vi "evaluate_SP_thcd401_ch1.vi"(7 "PID Range":cluster{"output high":dbl, "output low":dbl}={"output high"=10.0, "output low"=-10.0} {"output low" format="%.2f"; "output high" format="%.2f"}, 8 "ref_sp_ch1":refnum<vi>, 10 "F_org":dbl, 11 "control":dbl) -> (0 "status":u32(colorbox), 3 "F_new":dbl)   [LabVIEW 2019]
panel:
  out "lolo":dbl
  out "hihi":dbl
  out "lo":dbl=22.0
  out "hi":dbl=38.0
  in  "range_error":dbl=0.95
  in  "range_warn":dbl=0.9
  # "L/m"
  # "L/m"
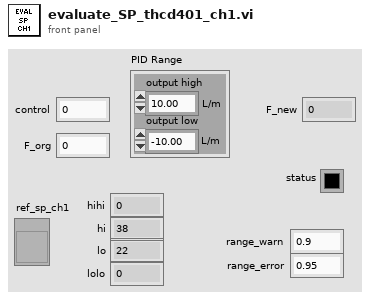
[diagram p1: front panel]
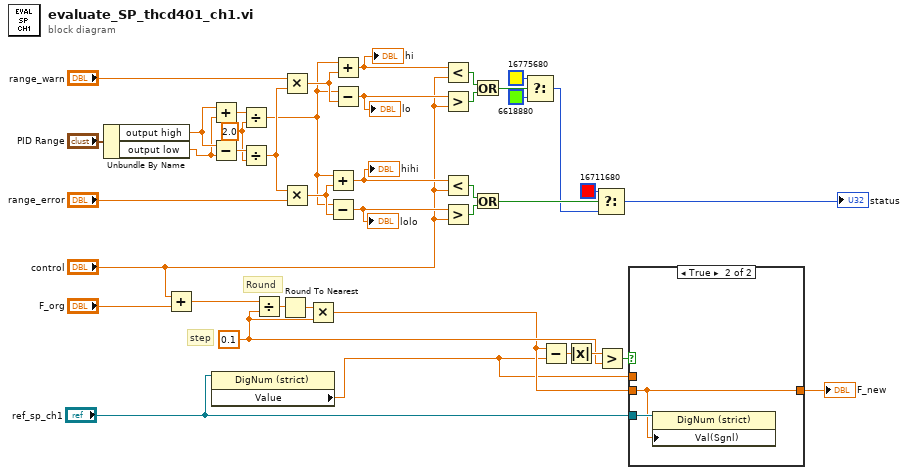
[diagram p0: block diagram]
diagram:
  w25 = 2.0 ("y")
  w34 = 0.1 ("y")
  # "Round"
  # "step"
  n1 = Unbundle By Name("PID Range") -> ("output high"=w20:dbl, "output low"=w19:dbl)
  n2 = Add(x="control", y="F_org") -> (x+y=w33:dbl)
  n3 = Add(x=w20, y=w19) -> (x+y=w27:dbl)
  n4 = Subtract(x=w20, y=w19) -> (x-y=w26:dbl)
  n5 = property class="DigNum (strict)"(reference="ref_sp_ch1") -> ("Value"=w3:dbl)  [unwired: 1 in, 2 out]
  n6 = Divide(x=w27, y=w25) -> (x/y=w10:dbl)
  n7 = Divide(x=w26, y=w25) -> (x/y=w11:dbl)
  n8 = Divide(x=w33, y=w34) -> (x/y=w36:dbl)
  n9 = Round To Nearest(number=w36) -> (nearest integer value=w35:dbl)
  n10 = Multiply(x="range_warn", y=w11) -> (x*y=w24:dbl)
  n11 = Multiply(x=w11, y="range_error") -> (x*y=w17:dbl)
  n12 = Multiply(x=w35, y=w34) -> (x*y=w9:dbl)
  n13 = Add(x=w10, y=w17) -> (x+y=w14:dbl)
  "hihi" <- w14
  n14 = Subtract(x=w10, y=w17) -> (x-y=w13:dbl)
  "lolo" <- w13
  n15 = Add(x=w10, y=w24) -> (x+y=w23:dbl)
  "hi" <- w23
  n16 = Subtract(x=w10, y=w24) -> (x-y=w22:dbl)
  "lo" <- w22
  n17 = Less?(x=w23, y="control") -> (x < y?=w29:bool)
  n18 = Greater?(x=w22, y="control") -> (0:w30:bool)
  n19 = Less?(x=w14, y="control") -> (x < y?=w15:bool)
  n20 = Greater?(x=w13, y="control") -> (0:w16:bool)
  n21 = Or(x=w29, y=w30) -> (x .or. y?=w28:bool)
  n22 = Or(x=w15, y=w16) -> (x .or. y?=w7:bool)
  n23 = Select(t=u32 16775680 ("alarm_status"), s=w28, f=u32 6618880 ("alarm_status")) -> (s? t:f=w6:u32)
  n24 = Subtract(x=w9, y=w3) -> (x-y=w40:dbl)
  n25 = Absolute Value(x=w40) -> (abs(x)=w39:dbl)
  n26 = Select(t=u32 16711680 ("alarm_status"), s=w7, f=w6) -> (s? t:f=→"status":u32)
  n27 = Greater?(x=w39, y=w34) -> (0:w38:bool)
  n28 = case shown="True" w38 {
    tunnel: "ref_sp_ch1" -> [_ w43]
    tunnel: w9 -> [_ w42]
    tunnel: [w41 w42] -> w4
    tunnel: w3 -> [w41 _]
    frame False {
    }
    frame True {
      n29 = property class="DigNum (strict)"(reference=w43, "Val(Sgnl)"=w42) -> ()  [unwired: 1 in, 2 out]
    }
  }
  "F_new" <- w4
